vi "LWXPS_PositionerCorrectorSR1ObserverAccelerationSet.vi"(5 "LabVIEW error IN":errorcluster, 6 "XPS Reference IN":refnum<k24>, 7 "Parameter C":dbl, 8 "Parameter B":dbl, 9 "Parameter A":dbl, 10 "Positioner Name":string) -> (0 "LabVIEW error OUT":errorcluster, 1 "XPS Error String":string, 2 "Returned error code":i32, 3 "XPS Reference OUT":refnum<k24>)   [LabVIEW 2014]
uses:
  D:/XPSQ8_LabView_Library/Development/Source/Dll/Newport.XPS.CommandInterface.dll
  Dll/Newport.XPS.CommandInterface.dll
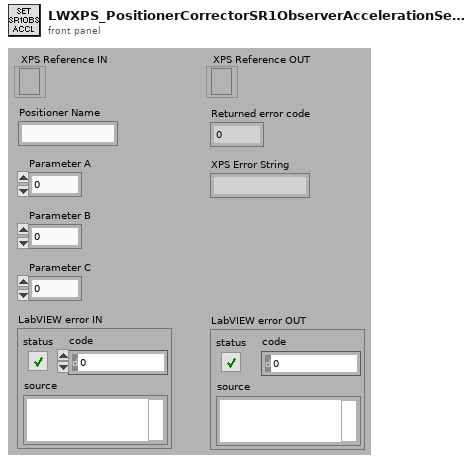
[diagram p1: front panel]
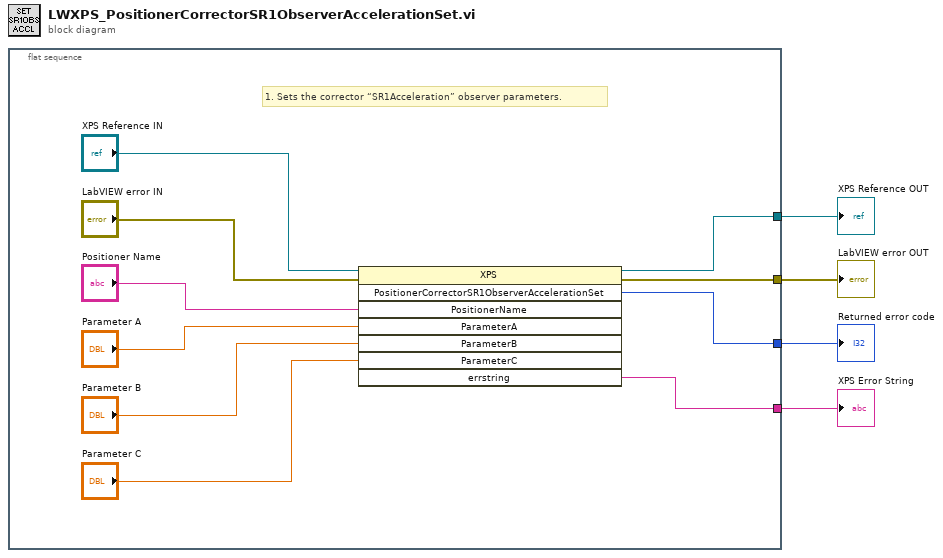
[diagram p0: block diagram]
diagram:
  n1 = flat-sequence {
    tunnel: [w10] -> w4
    tunnel: [w9] -> w3
    tunnel: [w11] -> w2
    tunnel: [w5] -> w1
    frame #0 {
      # "1. Sets the corrector “SR1Acceleration” observer parameters."
      n2 = invoke class="XPS" method="PositionerCorrectorSR1ObserverAccelerationSet"(reference="XPS Reference IN", error in="LabVIEW error IN", "PositionerName"="Positioner Name", "ParameterA"="Parameter A", "ParameterB"="Parameter B", "ParameterC"="Parameter C") -> (reference out=w10:refnum<k24>, error out=w9:errorcluster, "PositionerCorrectorSR1ObserverAccelerationSet"=w11:i32, "errstring"=w5:string)  [unwired: 2 in, 4 out]
    }
  }
  "XPS Error String" <- w1
  "XPS Reference OUT" <- w4
  "LabVIEW error OUT" <- w3
  "Returned error code" <- w2
